vi "WriteParams.vi"(8 "error in (no error)":errorcluster, 10 "Params":T1, 11 "reference in":refnum<class "Pgui_Obj.lvclass">) -> (0 "error out":errorcluster, 3 "reference out":refnum<class "Pgui_Obj.lvclass">)   [LabVIEW 2019, in "Pgui_Obj.lvclass"]
uses:
  Pgui_Obj.lvclass
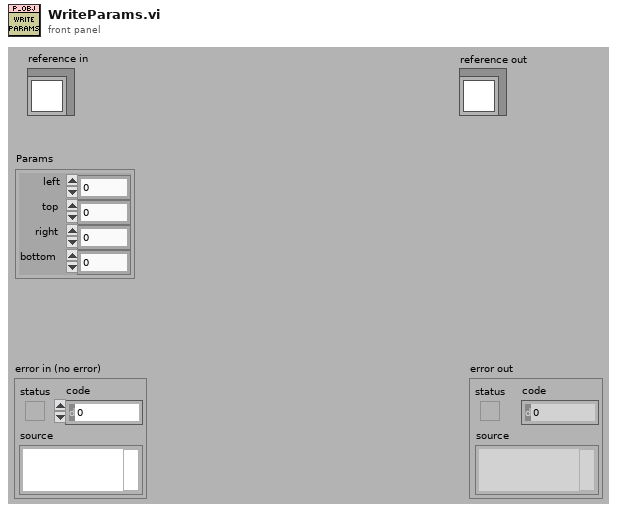
[diagram p1: front panel]
types:
  T1 = cluster{"left":i16, "top":i16, "right":i16, "bottom":i16}
  T2 = typedef "Pgui_Obj.lvclass/ObjectAttributes.ctl" = cluster{"Children":refnum<class "Pgui_Obj.lvclass">[], "Draw Instr":picture, "Params":cluster{"left":i16, "top":i16, "right":i16, "bottom":i16}, "Parent_Pgui_Obj":refnum<class "Pgui_Obj.lvclass">, "MouseOver":bool}
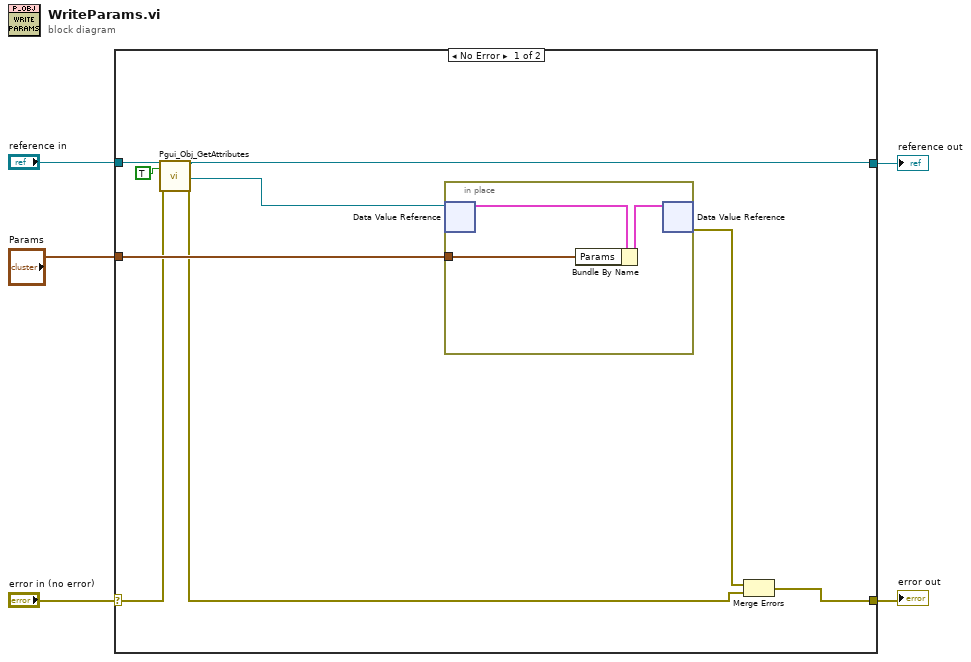
[diagram p0: block diagram]
diagram:
  n1 = case shown="No Error" "error in (no error)" {
    selector: "error in (no error)" -> [w8 w19]
    tunnel: [w12 w19] -> w4
    tunnel: [w10 w18] -> w2
    tunnel: "reference in" -> [w11 w18]
    tunnel: "Params" -> [w14 _]
    frame No Error {
      n2 = call "Pgui_Obj_GetAttributes.vi"("reference in"=w11, "OnlyGetDvrReference(False)"=TRUE, "error in (no error)"=w8) -> ("reference out"=w10:refnum<class "Pgui_Obj.lvclass">, "DataRef"=w9:refnum<data-value>, "error out"=w7:errorcluster)  [unwired: 13 in, 1 out]
      n3 = in-place {
        in-place-border: w14 -> [w17]
        n4 = in-place-dvr #1(w9) -> (w16:T2)  [unwired: 1 out]
        n5 = Bundle By Name(cluster=w16, "Params"=w17) -> (w15:T2)
        n6 = in-place-dvr #1(w15) -> (w13:errorcluster)  [unwired: 1 out]
      }
      n7 = Merge Errors(w13, w7) -> (w12:errorcluster)
    }
    frame Error {
    }
  }
  "error out" <- w4
  "reference out" <- w2
